vi "Alicat Server.vi"(0 "DVR In":refnum<data-value>) -> (14 "DVR out":refnum<data-value>)   [LabVIEW 2016]
uses:
  <vilib>/MSR Consulting, LLC/General Reuse/Session APIs/File Access/Config Data/Config Data.lvclass
  <vilib>/MSR Consulting, LLC/General Reuse/Session APIs/File Access/Config Data/Config Session.ctl
  <vilib>/MSR Consulting, LLC/General Reuse/Session APIs/_Session Fwk/Session - Root.lvclass
  <vilib>/MSR Consulting, LLC/Devices/Alicats/Alicat Device.lvclass
  <vilib>/Platform/TimedLoop/XDataNode/wakeup.ctl
  <vilib>/Platform/TimedLoop/XDataNode/XDNodeRunTimeDep.lvlib
  <vilib>/Platform/TimedLoop/XDataNode/nitl_modes.ctl
  <vilib>/Platform/TimedLoop/XDataNode/timing_clust.ctl
  <vilib>/Platform/TimedLoop/XDataNode/XDataNode.xnode
  <vilib>/MSR Consulting, LLC/General Reuse/Session APIs/Session Log/System Log.lvclass
  Data/Nicholas Data.lvclass
  <vilib>/MSR Consulting, LLC/Devices/Alicats/Data/Alicat Data.lvclass
  C:/Program Files (x86)/National Instruments/LabVIEW 2016/vi.lib/MSR Consulting, LLC/General Reuse/Session APIs/_Session Fwk/Session - Root.lvclass
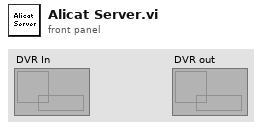
[diagram p1: front panel]
types:
  T1 = typedef "Config Data.lvclass/Config Session.ctl" = refnum<data-value>
  T2 = typedef "Session - Root.lvclass/Session Handle.ctl" = refnum<data-value>
  T3 = typedef "XDNodeRunTimeDep.lvlib/timing_clust.ctl" = cluster{"Expected End [f-1]":u64, "Actual End [f-1]":u64, "Finished Late? [f-1]":bool, "Expected End [i-1]":u64, "Actual End [i-1]":u64, "Finished Late? [i-1]":bool, "Expected Start [i]":u64, "Actual Start [i]":u64, "Expected Start [f]":u64, "Actual Start [f]":u64, "Source Name":string, "Structure Name":string, "Period":i64, "Deadline":i64, "Offset":i64, "Start":i64, "Priority":i32, "Timeout":i32, "Mode":T4, "Wakeup Reason":T5, "Error":errorcluster, "Source Type":string, "Secondary Source Type":string, "Global End Time":u64, "Global Start Time":u64, "Frame Duration":u64, "Iteration Duration":u64, "Assigned CPU":i32, "I/O Scan Engine Mode":u32}
  T4 = typedef "XDNodeRunTimeDep.lvlib/nitl_modes.ctl" = enum32{"No Change", "Process missed periods, maintain original phase", "Discard missed periods, maintain original phase", "Process missed periods, ignore original phase", "Discard missed periods, ignore original phase"}
  T5 = typedef "XDNodeRunTimeDep.lvlib/wakeup.ctl" = enum32{"Normal", "Aborted", "Asynchronous wakeup", "Timing source error", "Timed loop error", "Timeout"}
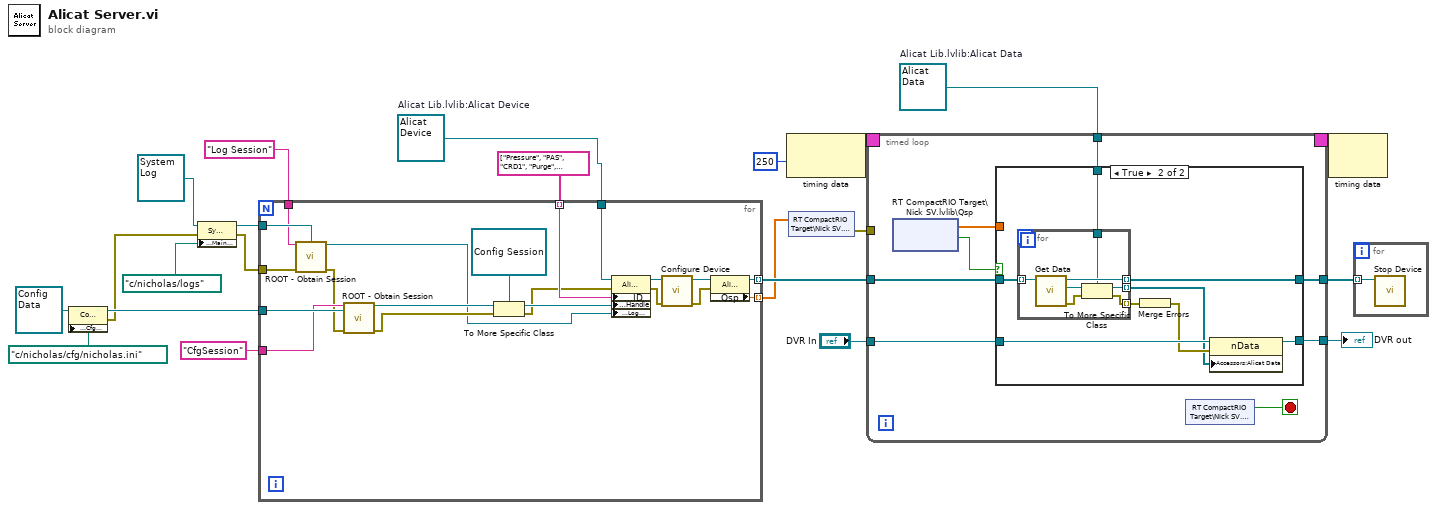
[diagram p0: block diagram]
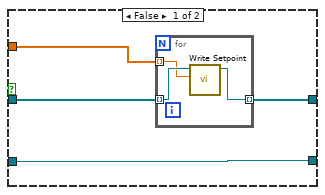
[diagram p2: hidden frame]
diagram:
  w1 = refnum<class "Alicat Data.lvclass"> refnum  # Alicat Lib.lvlib:Alicat Data
  w2 = refnum<class "Alicat Device.lvclass"> refnum  # Alicat Lib.lvlib:Alicat Device
  n1 = property class="Config Data"(reference=refnum<class "Config Data.lvclass"> refnum ("Config Data"), "Accessors:Cfg Path"=path "c:/nicholas/cfg/nicholas.ini" ("Cfg Path")) -> (reference out=w16:refnum<class "Config Data.lvclass">, error out=w6:errorcluster)  [unwired: 1 in]
  n2 = property class="Sys Log"(reference=refnum<class "System Log.lvclass"> refnum ("Sys Log"), error in=w6, "Accessors:Main Path"=path "c:/nicholas/logs" ("Main Path")) -> (reference out=w19:refnum<class "System Log.lvclass">, error out=w7:errorcluster)
  n3 = for {
    tunnel: w2 -> [w42]
    tunnel: w16 -> [w35]
    tunnel: "CfgSession" ("Session Name ()") -> [w34]
    tunnel: w19 -> [w41]
    tunnel: string[] ["Pressure", "PAS", "CRD1", "Purge", "Ozone", "AC6"] -> [w40] mode=indexing
    tunnel: [w27] -> w10 mode=indexing
    tunnel: w7 -> [w36]
    tunnel: "Log Session" ("Session Name ()") -> [w31]
    tunnel: [w25] -> w4 mode=indexing
    n4 = call <vilib>:"ROOT - Obtain Session.vi"("Session Name ()"=w31, "OBJ - Session"=w41, "error in (no error)"=w36) -> ("Session Handle"=w23:T2, "error out"=w30:errorcluster)  [unwired: 10 in, 1 out]
    n5 = call <vilib>:"ROOT - Obtain Session.vi"("Session Name ()"=w34, "OBJ - Session"=w35, "error in (no error)"=w30) -> ("Session Handle"=w33:T2, "error out"=w24:errorcluster)  [unwired: 10 in, 1 out]
    n6 = To More Specific Class(target class=T1 refnum ("Handle"), reference=w33, error in=w24) -> (specific class reference=w32:T1, error out=w29:errorcluster)
    n7 = property class="Alicat Device"(reference=w42, error in=w29, "Accessors:ID"=w40, "Accessors:Handle"=w32, "Accessors:Log Session"=w23) -> (reference out=w38:refnum<class "Alicat Device.lvclass">, error out=w37:errorcluster)
    n8 = call-dynamic "Configure Device.vi"("error in"=w37, "Alicat Device In"=w38) -> ("error out"=w26:errorcluster, "Alicat Device Out"=w28:refnum<class "Alicat Device.lvclass">)  [unwired: 6 in, 2 out]
    n9 = property class="Alicat Device"(reference=w28, error in=w26) -> (reference out=w27:refnum<class "Alicat Device.lvclass">, "Accessors:Qsp"=w25:dbl)  [unwired: 1 out]
  }
  n10 = node-c288(i64 250 ("Period")) -> (w22:T3)
  n11 = shared-variable "RT CompactRIO Target\\Nick SV.lvlib\\Qsp"(w4) -> (error out=w3:errorcluster)  [unwired: 1 in]
  n12 = timed-loop {
    tunnel: w10 -> [w50]
    tunnel: [w48] -> w11
    timing: w22 -> [_]
    timing-out: [_] -> w21
    tunnel: "DVR In" -> [w45]
    tunnel: [w44] -> w20
    tunnel: w3 -> [_]
    tunnel: w1 -> [w43]
    stop <- w49 stop-if-true
    n13 = shared-variable "RT CompactRIO Target\\Nick SV.lvlib\\Qsp"() -> (w46:sgl[], w47:bool)  [unwired: 2 in, 1 out]
    n14 = case shown="True" w47 {
      tunnel: w50 -> [w53 w65]
      tunnel: [w52 w64] -> w48
      tunnel: w46 -> [w54 _]
      tunnel: w45 -> [w51 w63]
      tunnel: [w51 w62] -> w44
      tunnel: w43 -> [_ w59]
      frame False {
        n15 = for {
          tunnel: w54 -> [w56] mode=indexing
          tunnel: w53 -> [w57] mode=indexing
          tunnel: [w55] -> w52 mode=indexing
          n16 = call <vilib>:"Write Setpoint.vi"("Setpoint"=w56, "Alicat Device in"=w57) -> ("Alicat Device out"=w55:refnum<class "Alicat Device.lvclass">)  [unwired: 7 in, 2 out]
        }
      }
      frame True {
        n17 = for {
          tunnel: w65 -> [w72] mode=indexing
          tunnel: [w71] -> w64 mode=indexing
          tunnel: w59 -> [w70]
          tunnel: [w68] -> w58 mode=indexing
          tunnel: [w66] -> w61 mode=indexing
          n18 = call-dynamic "Get Data.vi"("Alicat Device in"=w72) -> ("error out"=w67:errorcluster, "Data"=w69:refnum<class "Data.lvclass">, "Alicat Device out"=w71:refnum<class "Alicat Device.lvclass">)  [unwired: 8 in]
          n19 = To More Specific Class(target class=w70, reference=w69, error in=w67) -> (specific class reference=w68:refnum<class "Alicat Data.lvclass">, error out=w66:errorcluster)
        }
        n20 = Merge Errors(w61) -> (w60:errorcluster)
        n21 = property class="nData"(reference=w63, error in=w60, "Accessors:Alicat Data"=w58) -> (reference out=w62:refnum<data-value>)  [unwired: 1 out]
      }
    }
    n22 = shared-variable "RT CompactRIO Target\\Nick SV.lvlib\\Stop"() -> (w49:bool)  [unwired: 1 in, 1 out]
  }
  "DVR out" <- w20
  n23 = node-c288(w21) -> ()  [unwired: 1 out]
  n24 = for {
    tunnel: w11 -> [w75] mode=indexing
    n25 = call-dynamic "Stop Device.vi"("Alicat Device in"=w75) -> ()  [unwired: 9 in, 2 out]
  }
